vi "TcA01-010_GarbageCollectorWithSameOwner.vi"(1 "Input buffer":T3="1", 3 "Invocation info":T2, 5 "error in (no error)":errorcluster, 6 "Add log to result?":bool) -> (16 "Test Data":T1 {"Numeric Measurement" format="%.2f"}, 19 "error out":errorcluster)   [LabVIEW 2020]
doc: "Test case template."
uses:
  Shared/Support_InputBuffer.ctl
  Shared/Support_InvocationInfo.ctl
  Shared/Support_TestData.ctl
  <vilib>/addons/_AddQ/G#Object/G#Object.lvclass
  TestClasses/G#SubClass1_class/G#SubClass1.lvclass
panel:
  in  "Test name":string="TcA01-010 Garbage collector with same owner"
  out "Test result":bool
  out "Result":string
  # "Verify that garbage collector with different owner works."
  # "Sub test case"
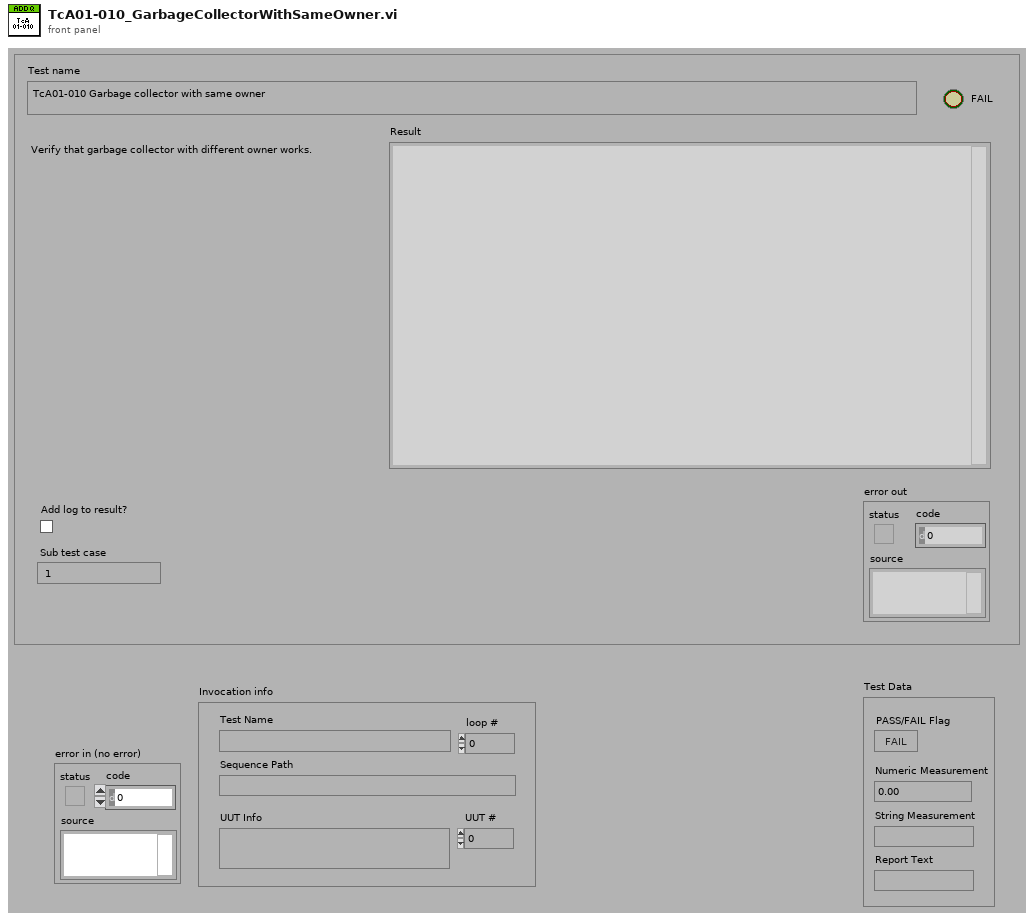
[diagram p1: front panel]
types:
  T1 = typedef "Support_TestData.ctl" = cluster{"PASS/FAIL Flag":bool, "Numeric Measurement":dbl, "String Measurement":string, "Report Text":string}
  T2 = typedef "Support_InvocationInfo.ctl" = cluster{"UUT #":i32, "loop #":i32, "UUT Info":string, "Test Name":string, "Sequence Path":path}
  T3 = typedef "Support_InputBuffer.ctl" = string
  T4 = typedef "Support_ResultType.ctl" = cluster{"Pass":bool, "Comment":string, "MeasurementValue":dbl}
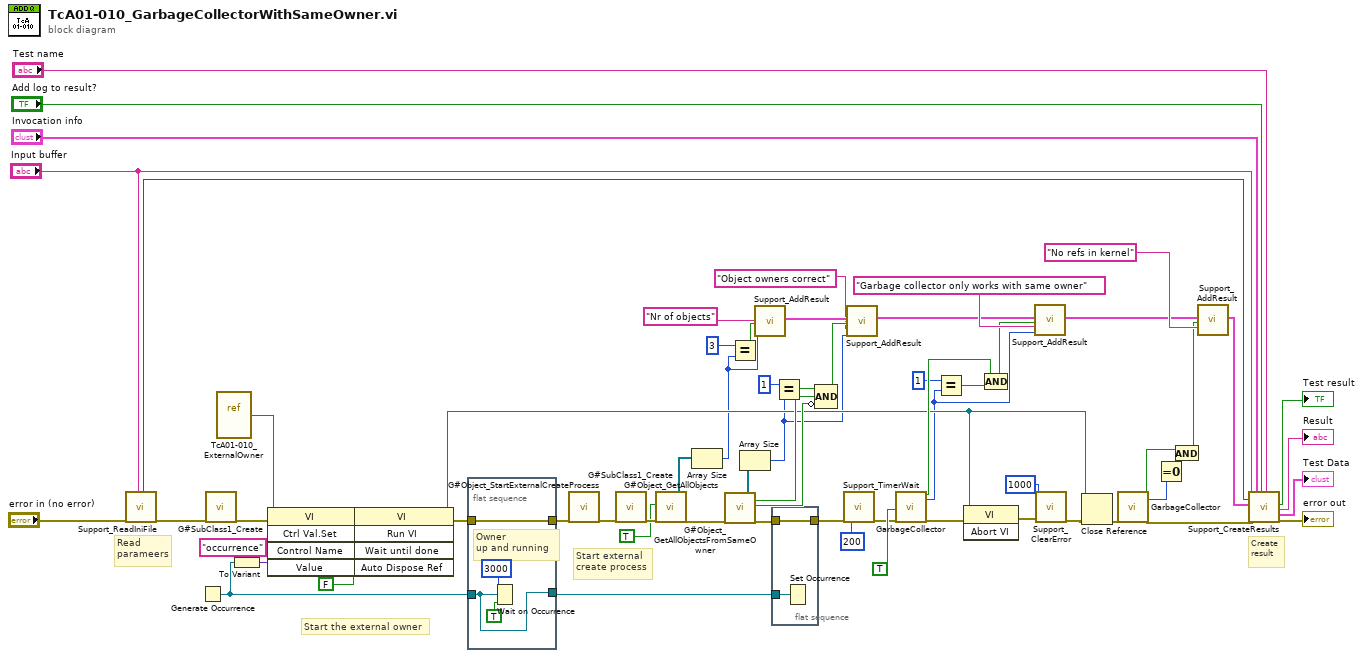
[diagram p0: block diagram]
diagram:
  # "Start external\ncreate process"
  # "Start the external owner"
  # "Read\nparameers"
  # "Create\nresult"
  n1 = call "Support_ReadIniFile.vi"("error in (no error)"="error in (no error)", "Sub test case"="Input buffer") -> ("Timer start"=w55:u32, "error out"=w46:errorcluster)  [unwired: 10 in, 6 out]
  n2 = Generate Occurrence() -> (w7:refnum<k4>)
  n3 = call "G#SubClass1_Create.vi"("error in (no error)"=w46) -> ("error out"=w44:errorcluster)  [unwired: 16 in, 2 out]
  n4 = vi-ref "TcA01-010_ExternalOwner.vi"() -> (w43:refnum<vi>)
  n5 = To Variant(anything=w7) -> (Variant=w41:variant)
  n6 = invoke class="VI" method="Ctrl Val.Set"(reference=w43, error in=w44, "Control Name"="occurrence", "Value"=w41) -> (reference out=w40:refnum<vi>, error out=w39:errorcluster)  [unwired: 1 in, 3 out]
  n7 = invoke class="VI" method="Run VI"(reference=w40, error in=w39, "Wait until done"=FALSE ("Wait Until Done")) -> (reference out=w16:refnum<vi>, error out=w6:errorcluster)  [unwired: 2 in, 3 out]
  n8 = flat-sequence {
    tunnel: w7 -> [w67]
    tunnel: w6 -> [w68]
    tunnel: [w68] -> w5
    tunnel: [w67] -> w4
    frame #0 {
      # "Owner\nup and running"
      n9 = Wait on Occurrence(1:TRUE ("ignore previous (T)"), 2:w67, 3:3000 ("ms timeout (-1)")) -> ()  [unwired: 1 out]
    }
  }
  n10 = call <vilib>:"G#Object_StartExternalCreateProcess.vi"("error in (no error)"=w5) -> ("error out"=w45:errorcluster)  [unwired: 18 in]
  n11 = call "G#SubClass1_Create.vi"("error in (no error)"=w45) -> ("error out"=w34:errorcluster)  [unwired: 16 in, 2 out]
  n12 = call <vilib>:"G#Object_GetAllObjects.vi"("only refs (F)"=TRUE ("only refs"), "error in (no error)"=w34) -> ("all refs"=w32:refnum<class "G#Object.lvclass">[], "error out"=w31:errorcluster)  [unwired: 14 in, 2 out]
  n13 = Array Size(array=w32) -> (size(s)=w11:i32)
  n14 = call <vilib>:"G#Object_GetAllObjectsFromSameOwner.vi"("error in (no error)"=w31) -> ("all refs"=w30:refnum<class "G#Object.lvclass">[], "external creator process owns"=w23:bool, "no other owners"=w24:bool, "error out"=w3:errorcluster)  [unwired: 15 in]
  n15 = Equal?(x=3, y=w11) -> (x = y?=w29:bool)
  n16 = Array Size(array=w30) -> (size(s)=w10:i32)
  n17 = call "Support_AddResult.vi"("Pass"=w29, "Comment"="Nr of objects", "MeasurementValue"=w11) -> ("Results out"=w27:T4[])  [unwired: 16 in]
  n18 = flat-sequence {
    tunnel: w4 -> [w72]
    tunnel: w3 -> [w71]
    tunnel: [w71] -> w37
    frame #0 {
      n19 = Set Occurrence(w72) -> ()
    }
  }
  n20 = Equal?(x=1, y=w10) -> (x = y?=w25:bool)
  n21 = Compound Arithmetic op=AND(w25, w23, invert w24) -> (w22:bool)
  n22 = call "Support_TimerWait.vi"("error in (no error)"=w37, "milliseconds to wait"=u32 200) -> ("error out"=w2:errorcluster)  [unwired: 17 in]
  n23 = call "Support_AddResult.vi"("Results in"=w27, "Pass"=w22, "Comment"="Object owners correct", "MeasurementValue"=w10) -> ("Results out"=w20:T4[])  [unwired: 15 in]
  n24 = call <vilib>:"GarbageCollector.vi"("only from same owner as caller? (T)"=TRUE ("only from same owner as caller?"), "error in (no error)"=w2) -> ("OK"=w18:bool, "# of objects killed"=w9:i32, "error out"=w1:errorcluster)  [unwired: 15 in]
  n25 = Equal?(x=1, y=w9) -> (x = y?=w19:bool)
  n26 = invoke class="VI" method="Abort VI"(reference=w16, error in=w1) -> (error out=w14:errorcluster)  [unwired: 1 in, 2 out]
  n27 = Compound Arithmetic op=AND(w18, w19) -> (w15:bool)
  n28 = call "Support_AddResult.vi"("Results in"=w20, "Pass"=w15, "Comment"="Garbage collector only works with same owner", "MeasurementValue"=w9) -> ("Results out"=w47:T4[])  [unwired: 15 in]
  n29 = call "Support_ClearError.vi"("code"=1000, "error in (no error)"=w14) -> ("error out"=w13:errorcluster)  [unwired: 16 in, 1 out]
  n30 = Close Reference(reference=w16, error in (no error)=w13) -> (error out=w35:errorcluster)
  n31 = call <vilib>:"GarbageCollector.vi"("error in (no error)"=w35) -> ("OK"=w51:bool, "# of objects killed"=w49:i32, "error out"=w54:errorcluster)  [unwired: 16 in]
  n32 = Equal To 0?(x=w49) -> (x = 0?=w50:bool)
  n33 = And(x=w51, y=w50) -> (x .and. y?=w48:bool)
  n34 = call "Support_AddResult.vi"("Results in"=w47, "Pass"=w48, "Comment"="No refs in kernel") -> ("Results out"=w53:T4[])  [unwired: 16 in]
  n35 = call "Support_CreateResults.vi"("Sub test case"="Input buffer", "Timer start"=w55, "Results"=w53, "error in (no error)"=w54, "Invocation info"="Invocation info", "Add log to result?"="Add log to result?", "Test name"="Test name") -> ("Pass/fail flag"=→"Test result":bool, "Result"=→"Result":string, "Test Data"=→"Test Data":T1, "error out"=→"error out":errorcluster)  [unwired: 9 in]
